vi "UserInterface.vi"(8 "error in (no error)":errorcluster, 11 "View in":refnum<class "View.lvclass">) -> (0 "error out":errorcluster, 3 "View out":refnum<class "View.lvclass">)   [LabVIEW 2020, in "UIContainer.lvlib" / "View.lvclass"]
uses:
  View.lvclass
  View.lvclass/View.ctl
  Controller/Controller.lvclass
panel:
  in  "Settings Button":bool
  in  "Home Button":bool
  # "Container User Interface"
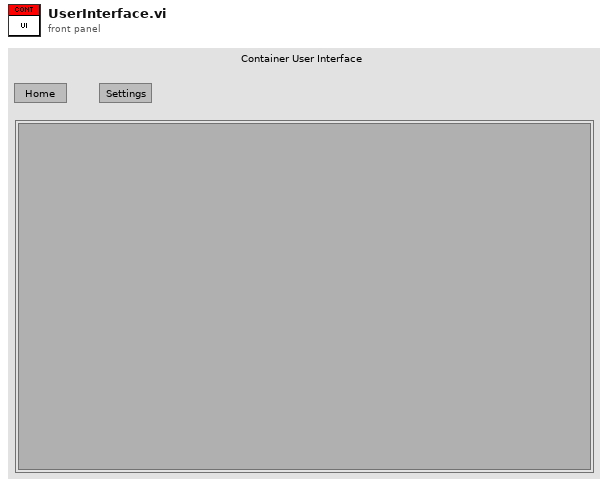
[diagram p1: front panel]
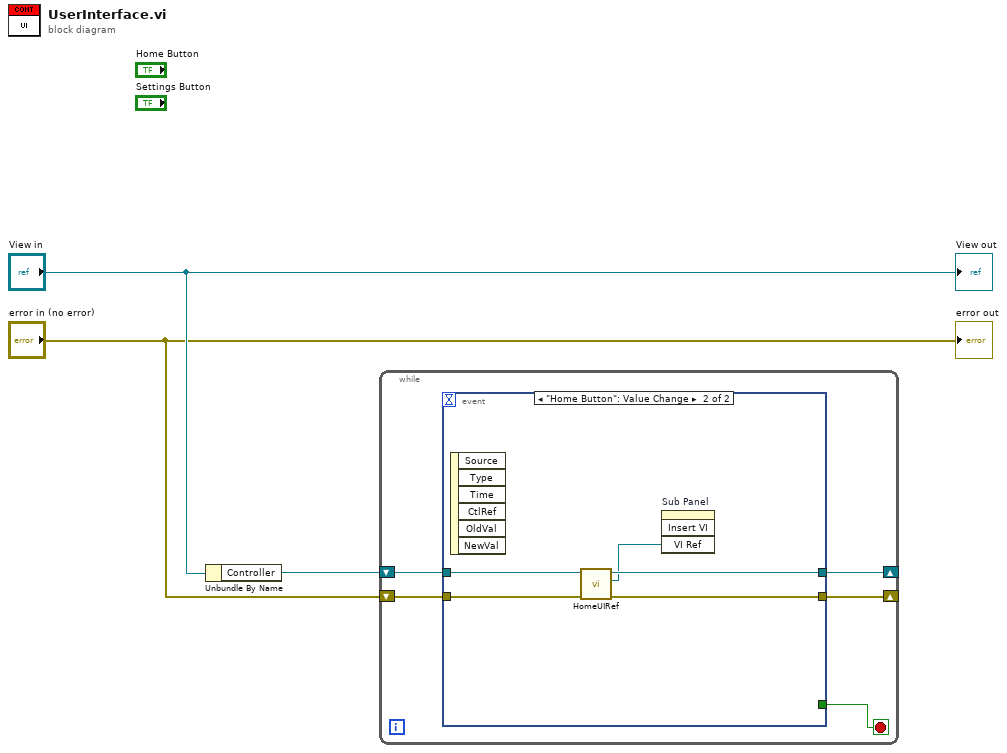
[diagram p0: block diagram]
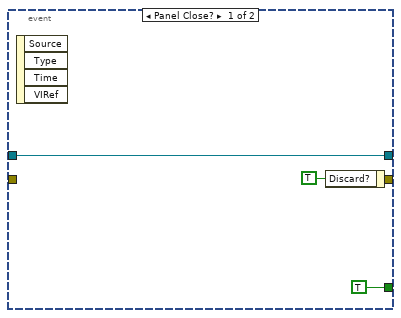
[diagram p2: hidden frame]
diagram:
  n1 = Unbundle By Name("View in") -> ("Controller"=w2:refnum<class "Controller.lvclass">)
  n2 = while {
    shift-right: [w6] -> _
    shift-left: w2 -> [w7]
    shift-right: [w5] -> _
    shift-left: "error in (no error)" -> [w4]
    stop <- w8 stop-if-true
    n3 = event shown="[1] \"Home Button\": Value Change" {
      selector: _ -> [_ _]
      dyn-events: _ -> [_ _]
      timeout: _ -> [_ _]
      tunnel: [TRUE _] -> w8
      tunnel: w7 -> [w9 w16]
      tunnel: [w9 w15] -> w6
      tunnel: [_ w14] -> w5
      tunnel: w4 -> [_ w13]
      event Panel Close? {
        n4 = event-data() -> ()  [unwired: 1 in, 4 out]
        n5 = event-data("Discard?"=TRUE) -> ()  [unwired: 1 in, 1 out]
      }
      event "Home Button": Value Change {
        n6 = event-data() -> ()  [unwired: 1 in, 6 out]
        n7 = call "HomeUIRef.vi"("error in (no error)"=w13, "Controller in"=w16) -> ("error out"=w14:errorcluster, "VIRef"=w12:refnum<vi>, "Controller out"=w15:refnum<class "Controller.lvclass">)  [unwired: 7 in]
        n8 = invoke on="Sub Panel" class="SubPnl" method="Insert VI"("VI Ref"=w12) -> ()  [unwired: 3 in, 4 out]
      }
    }
  }
  "error out" <- "error in (no error)"
  "View out" <- "View in"
